vi "Read Serial Setting.vi"(8 "error in (no error)":errorcluster, 11 "Device Parameter":string[][](array[string])) -> (0 "error out":errorcluster, 3 "Serial Parameetr":T1={"VISA resource name"="", "baud rate (9600)"=9600, "data bits (8)"=8, "parity (0:none)"=enum."None", "stop bits (10: 1 bit)"=10, "flow control (0:none)"=0, "termination char\n(0xA = '\\n' = LF) "=10, "Enable Termination\nChar (T)"=TRUE, "timeout (10sec)"=10000} {"flow control (0:none)" items=["None", "XON/XOFF", "RTS/CTS", "XON/XOFF & RTS/CTS", "DTR/DSR", "XON/XOFF & DTR/DSR"]; "stop bits (10: 1 bit)" items=["1.0"=10, "1.5"=15, "2.0"=20]; "termination char\n(0xA = '\\n' = LF)" format="%.0x"; "data bits (8)" min=5 max=8 step=1})   [LabVIEW 2021, in "Serial Hardware.lvlib"]
uses:
  Serial Parameter.ctl
  Serial Hardware.lvlib
  User Interface/User Interface.lvlib
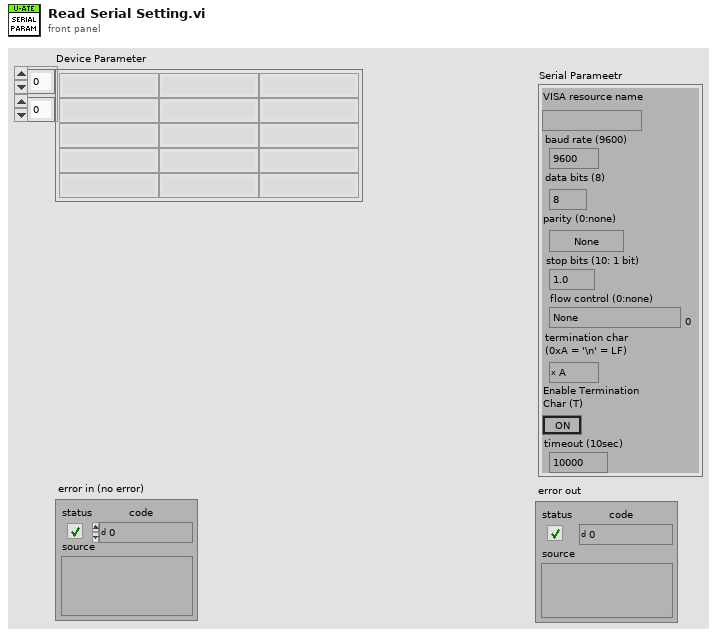
[diagram p1: front panel]
types:
  T1 = typedef "Serial Hardware.lvlib/Serial Parameter.ctl" = cluster{"VISA resource name":refnum<visa-resource-name>, "baud rate (9600)":u32, "data bits (8)":u16, "parity (0:none)":enum16{"None", "Odd", "Even", "Mark", "Space"}, "stop bits (10: 1 bit)":u16, "flow control (0:none)":u16, "termination char\n(0xA = '\\n' = LF) ":u8, "Enable Termination\nChar (T)":bool, "timeout (10sec)":u32}
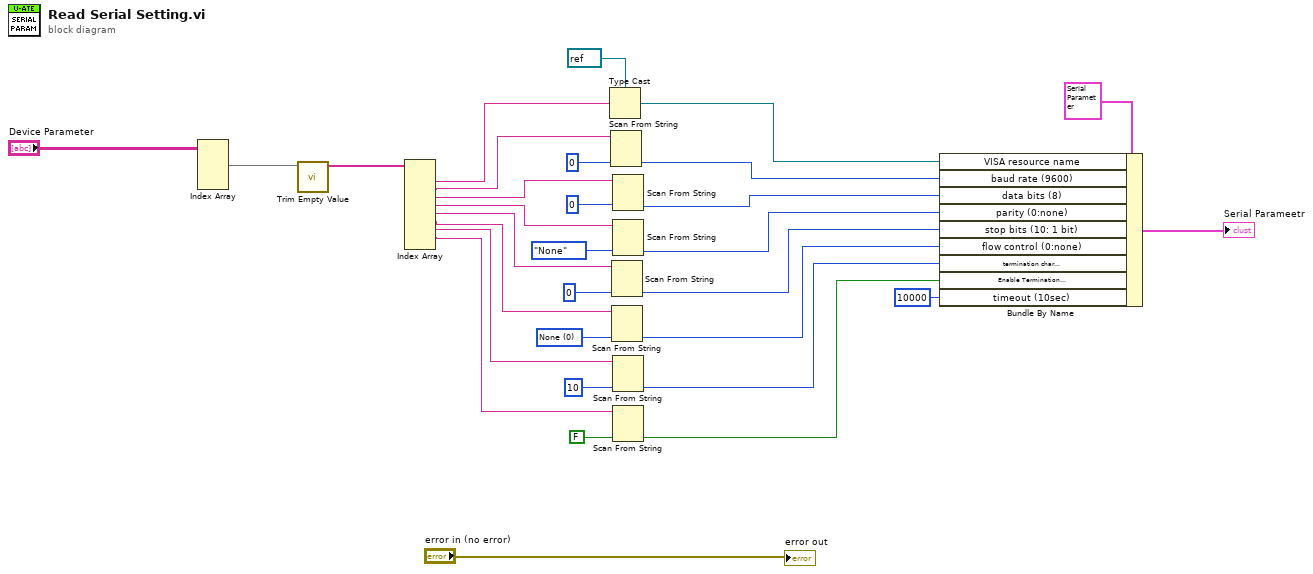
[diagram p0: block diagram]
diagram:
  w10 = u16 0 items=["None", "XON/XOFF", "RTS/CTS", "XON/XOFF & RTS/CTS", "DTR/DSR", "XON/XOFF & DTR/DSR"] ("flow control (0:none)")
  n1 = Index Array(array="Device Parameter") -> (element #1=w29:string[])  [unwired: 4 in, 1 out]
  n2 = call "Trim Empty Value.vi"("Data In"=w29) -> ("Data Out"=w28:string[])  [unwired: 10 in]
  n3 = Index Array(array=w28) -> (element #1=w26:string, element #2=w23:string, element #3=w20:string, element #4=w17:string, element #5=w14:string, element #6=w11:string, element #7=w8:string, element #8=w4:string)  [unwired: 9 in, 1 out]
  n4 = Type Cast(type=refnum<visa-resource-name> refnum ("VISA resource name"), x=w26) -> (*(type *) &x=w24:refnum<visa-resource-name>)
  n5 = Scan From String(input string=w23, default 1=u32 0 ("baud rate (9600)")) -> (output 1=w21:u32)  [unwired: 3 in, 3 out]
  n6 = Scan From String(input string=w14, default 1=u16 0 ("stop bits (10: 1 bit)")) -> (output 1=w12:u16)  [unwired: 3 in, 3 out]
  n7 = Scan From String(input string=w11, default 1=w10) -> (output 1=w9:u16)  [unwired: 3 in, 3 out]
  n8 = Scan From String(input string=w20, default 1=u16 0 ("data bits (8)")) -> (output 1=w18:u16)  [unwired: 3 in, 3 out]
  n9 = Scan From String(input string=w17, default 1=enum16{"None", "Odd", "Even", "Mark", "Space"}."None" ("parity (0:none)")) -> (output 1=w15:enum16{"None", "Odd", "Even", "Mark", "Space"})  [unwired: 3 in, 3 out]
  n10 = Scan From String(input string=w8, default 1=u8 10 ("termination char\n(0xA = '\\n' = LF)")) -> (output 1=w6:u8)  [unwired: 3 in, 3 out]
  n11 = Scan From String(input string=w4, default 1=FALSE) -> (output 1=w3:bool)  [unwired: 3 in, 3 out]
  n12 = Bundle By Name(cluster=T1 {"VISA resource name"="", "baud rate (9600)"=9600, "data bits (8)"=8, "parity (0:none)"=enum."None", "stop bits (10: 1 bit)"=10, "flow control (0:none)"=0, "termination char\n(0xA = '\\n' = LF) "=10, "Enable Termination\nChar (T)"=TRUE, "timeout (10sec)"=10000}, "VISA resource name"=w24, "baud rate (9600)"=w21, "data bits (8)"=w18, "parity (0:none)"=w15, "stop bits (10: 1 bit)"=w12, "flow control (0:none)"=w9, "termination char\n(0xA = '\\n' = LF)"=w6, "Enable Termination\nChar (T)"=w3, "timeout (10sec)"=u32 10000) -> (→"Serial Parameetr":T1)
  "error out" <- "error in (no error)"
